vi "SQL Server Info.vi"() -> (0 "SQL Server Info":T2={"Port"=3306, "IP Address"="192.168.10.248", "Authentication"={"User"="loasis", "Password"="dat+l0sim", "Database"="loasis"}})   [LabVIEW 2011]
uses:
  shared programs/MySQL/typedefs/mysql_authentication.ctl
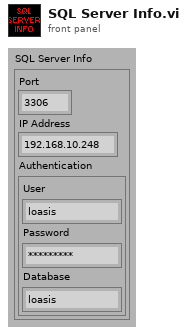
[diagram p1: front panel]
types:
  T1 = typedef "mysql_authentication.ctl" = cluster{"User":string, "Password":string, "Database":string}
  T2 = cluster{"Port":u16, "IP Address":string, "Authentication":T1}
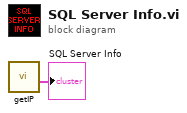
[diagram p0: block diagram]
diagram:
  n1 = call "getIP.vi"() -> ("SQL Server Info"=→"SQL Server Info":T2)  [unwired: 4 in, 4 out]
